vi "CA_for work.vi"() -> (4 "input ports":u8[](array[numeric]), 6 "modified output ports":u8[](array[numeric]), 8 "Clear ALG input array":cluster{i32, "Value":string, i32}[](array[cluster]), 10 "ALG output array":cluster{i32, "Value":string, i32}[](array[cluster]))   [LabVIEW 2012]
uses:
  canon_dll.dll
panel:
  out "states":cluster{u32, u8}[][](array[cluster])
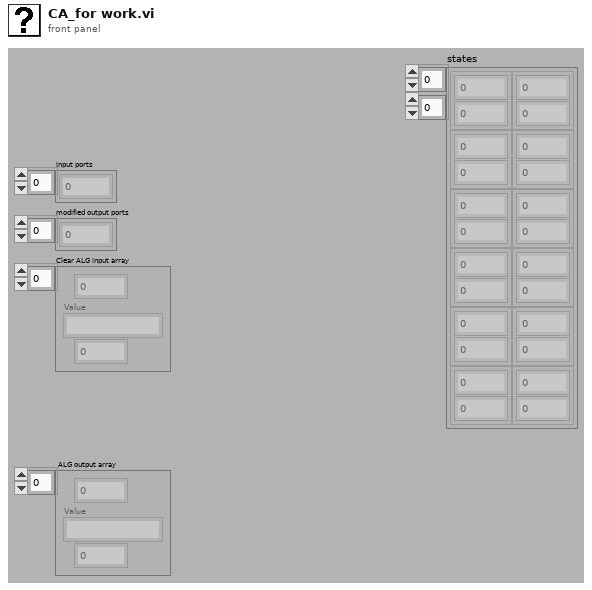
[diagram p1: front panel]
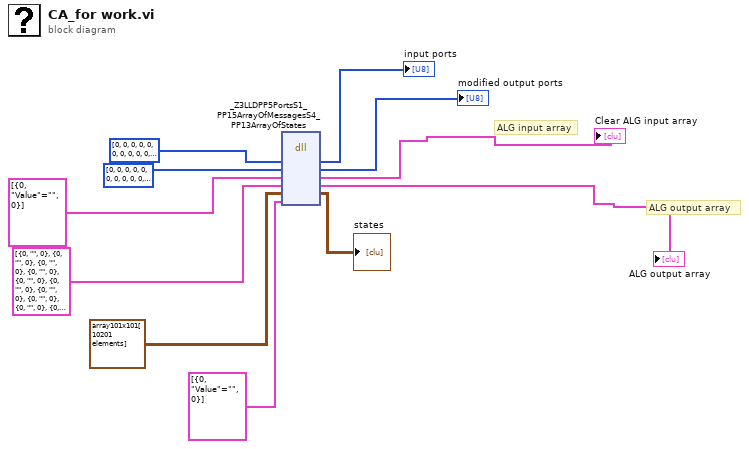
[diagram p0: block diagram]
diagram:
  # "ALG input array"
  # "ALG output array"
  n1 = dll-call lib="C:/Users/HP/Documents/NSU/DIPLOMA WORK/Aspirantura/Nonius/New debug prog/libs testing/canon_dll.dll" fn="_Z3LLDPP5PortsS1_PP15ArrayOfMessagesS4_PP13ArrayOfStates" label="AY"("input"=u8[] [0, 0, 0, 0, 0, 0, 0, 0, 0, 0, 0, 0, 0, 0, 0, 0, 0, 0, 0, 0, 0] ("init input ports"), "output"=u8[] [0, 0, 0, 0, 0, 0, 0, 0, 0, 0, 0, 0, 0, 0, 0, 0, 0, 0, 0, 0, 0], "msg_inp"=cluster{i32, "Value":string, i32}[] [{0, "Value"="", 0}] ("input ALG msg array"), "msg_inp"=cluster{i32, "Value":string, i32}[] [{0, "Value"="", 0}, {0, "Value"="", 0}, {0, "Value"="", 0}, {0, "Value"="", 0}, {0, "Value"="", 0}, {0, "Value"="", 0}, {0, "Value"="", 0}, {0, "Value"="", 0}, {0, "Value"="", 0}, {0, "Value"="", 0}, {0, "Value"="", 0}, {0, "Value"="", 0}, {0, "Value"="", 0}, {0, "Value"="", 0}, {0, "Value"="", 0}, {0, "Value"="", 0}, {0, "Value"="", 0}, {0, "Value"="", 0}, {0, "Value"="", 0}, {0, "Value"="", 0}, {0, "Value"="", 0}] ("Output ALG msg array"), "states"=cluster{u32, u8}[][] array101x101[10201 elements] ("Alg states"), "voc_msg"=cluster{i32, "Value":string, i32}[] [{0, "Value"="", 0}] ("VOC output msg CASHE")) -> ("input"=→"input ports":u8[], "output"=→"modified output ports":u8[], "msg_inp"=→"Clear ALG input array":cluster{i32, "Value":string, i32}[], "msg_inp"=→"ALG output array":cluster{i32, "Value":string, i32}[], "states"=→"states":cluster{u32, u8}[][])  [unwired: 5 in, 2 out]
